vi "Read Number of Lines.vi"(8 "error in (no error)":errorcluster, 11 "Iterative Dispense in":refnum<class "Iterative Dispense.lvclass">) -> (0 "error out":errorcluster, 2 "Number of Lines":i32, 3 "Iterative Dispense out":refnum<class "Iterative Dispense.lvclass">)   [LabVIEW 2020, in "Iterative Dispense.lvclass"]
uses:
  Iterative Dispense.lvclass
  Iterative Dispense.lvclass/Iterative Dispense.ctl
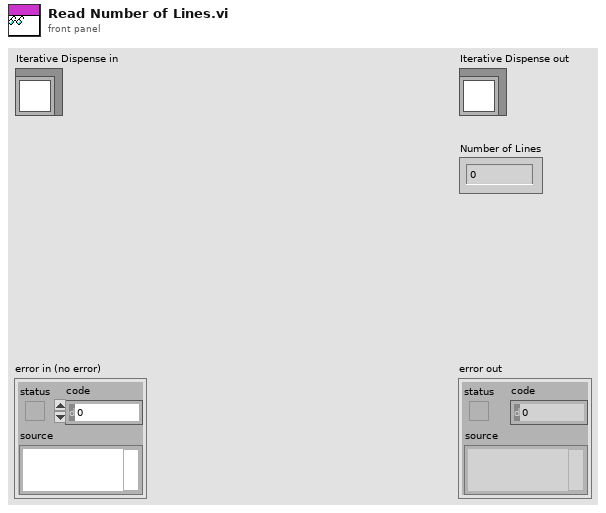
[diagram p1: front panel]
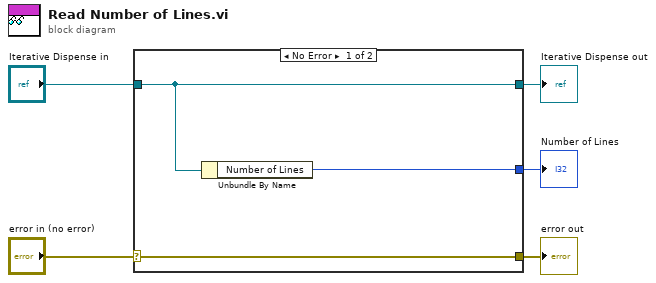
[diagram p0: block diagram]
diagram:
  n1 = case shown="No Error" "error in (no error)" {
    selector: "error in (no error)" -> [w8 w9]
    tunnel: [w8 w9] -> w4
    tunnel: [w7 w10] -> w2
    tunnel: "Iterative Dispense in" -> [w7 w10]
    tunnel: [w6 _] -> w1
    frame No Error {
      n2 = Unbundle By Name(w7) -> ("Number of Lines"=w6:i32)
    }
    frame Error {
    }
  }
  "error out" <- w4
  "Iterative Dispense out" <- w2
  "Number of Lines" <- w1
